vi "teleop_Moteur_Independant.vi"(11 "SwerveDrive":T1) -> ()   [LabVIEW 2018]
doc: "Les axes X and Y sont les deux axes qui font avancer le robot. X est horizontal et Y vertical selon le pilote.\nL'axez Z est l'axe qui permet au pilote de tourner en avançant dans une direction.\nLes boutons gauche et droite permettent au robot de tourner sur lui-même vers la gauche ou vers la droite selon quel bouton est actif.\n\nLe code vérifie que les roues sont dans le bon angle avant de faire avancer le robot."
uses:
  SwerveDrive.ctl
  <vilib>/addons/control/pid/pid.llb/PID (DBL).vi
  MyGlobal.vi
  <vilib>/addons/control/pid/NI_PID_pid.lvlib
panel:
  out "OUTPUT avant gauche":dbl format="%.2f"
  out "result":bool
  out "Encodeur angle arriere droite":bool
  out "Encodeur angle arriere gauche":bool
  out "Encodeur angle arriere droite":dbl
  out "Encodeur angle arriere gauche":dbl
  out "Encodeur angle avant droite":bool
  out "Encodeur angle avant gauche":bool
  out "angle roues":dbl
  out "Encodeur angle avant droite":dbl
  out "Encodeur angle avant gauche":dbl
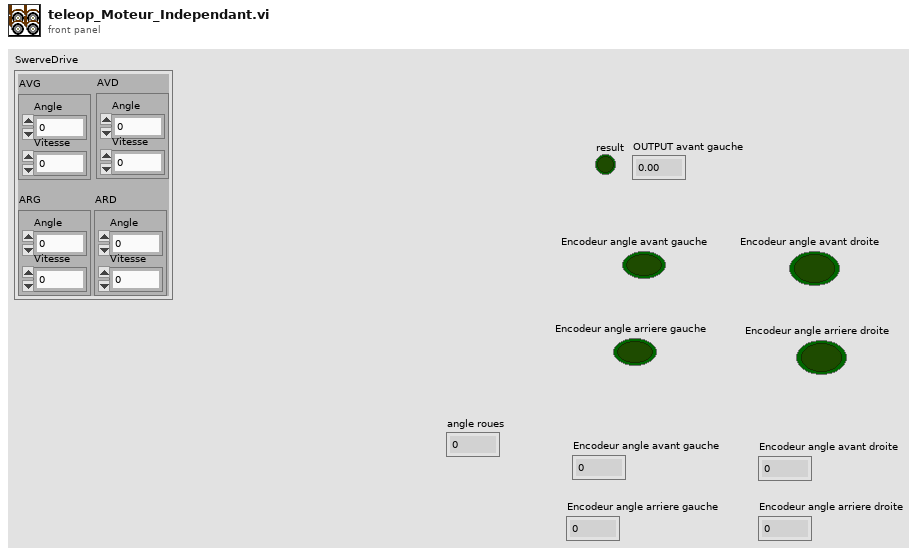
[diagram p1: front panel]
types:
  T1 = typedef "SwerveDrive.ctl" = cluster{"AVD":cluster{"Angle":dbl, "Vitesse":dbl}, "AVG":cluster{"Angle":dbl, "Vitesse":dbl}, "ARG":cluster{"Angle":dbl, "Vitesse":dbl}, "ARD":cluster{"Angle":dbl, "Vitesse":dbl}}
  T2 = cluster{"proportional gain (Kc)":dbl, "integral time (Ti, min)":dbl, "derivative time (Td, min)":dbl}
  T3 = typedef "Drivetype.ctl" = enum16{"4 vitesse", "1 vitesse"}
  T4 = typedef "WPI_MotorControlDeviceRef.ctl" = cluster{"DeviceStatus":errorcluster, "Type":T5, "PWM":cluster{"PWM Channel":T6, "DeadBand":T7}, "CAN":cluster{"Device Number":u8, "SetOutput VI Ref":variant, "GetOutput VI Ref":variant, "Enable VI Ref":variant, "Disable VI Ref":variant, "Data":variant}, "Invert":bool, "DIO PWM":cluster{"PWM \"Enable\" Channel":T6, "DIOChannel":T8, "PWM Rate":dbl}}
  T5 = typedef "WPI_MotorControlType.ctl" = enum16{"PWM", "CAN", "DIO PWM"}
  T6 = typedef "FPGA_DIOPWMChannel.ctl" = enum8{"PWM 0", "PWM 1", "PWM 2", "PWM 3", "PWM 4", "PWM 5", "PWM 6", "PWM 7", "PWM 8", "PWM 9", "PWM MXP 0", "PWM MXP 1", "PWM MXP 2", "PWM MXP 3", "PWM MXP 4", "PWM MXP 5", "PWM MXP 6", "PWM MXP 7", "PWM MXP 8", "PWM MXP 9", "Invalid"}
  T7 = typedef "WPI_PWMDeadband.ctl" = cluster{"Name":string, "maxPositivePwm":i32, "minPositivePwm":i32, "centerPwm":i32, "maxNegativePwm":i32, "minNegativePwm":i32, "angularRange":u16}
  T8 = typedef "FPGA_DIOChannel.ctl" = enum8{"DIO 0", "DIO 1", "DIO 2", "DIO 3", "DIO 4", "DIO 5", "DIO 6", "DIO 7", "DIO 8", "DIO 9", "DIO MXP 0", "DIO MXP 1", "DIO MXP 2", "DIO MXP 3", "DIO MXP 4", "DIO MXP 5", "DIO MXP 6", "DIO MXP 7", "DIO MXP 8", "DIO MXP 9", "DIO MXP 10", "DIO MXP 11", "DIO MXP 12", "DIO MXP 13", "DIO MXP 14", "DIO MXP 15", "SPI Port CS1", "SPI Port CS2", "SPI Port CS3", "SPI Port MISO", "SPI Port MOSI", "Invalid"}
  T9 = typedef "WPI_EncoderDevRef.ctl" = cluster{"DevStatus":errorcluster, "EncoderIndex":T10, "CounterIndex":T11, "DistancePerCount":dbl, "Decoding Type":T12}
  T10 = typedef "FPGA_EncoderIdx.ctl" = enum8{"Enc 0", "Enc 1", "Enc 2", "Enc 3", "Enc 4", "Enc 5", "Enc 6", "Enc 7", "Invalid"}
  T11 = typedef "FPGA_CounterCtrSystemIndex.ctl" = enum8{"Ctr 0", "Ctr 1", "Ctr 2", "Ctr 3", "Ctr 4", "Ctr 5", "Ctr 6", "Ctr 7", "Invalid"}
  T12 = typedef "WPI_EncoderType.ctl" = enum16{"1x", "2x", "4x"}
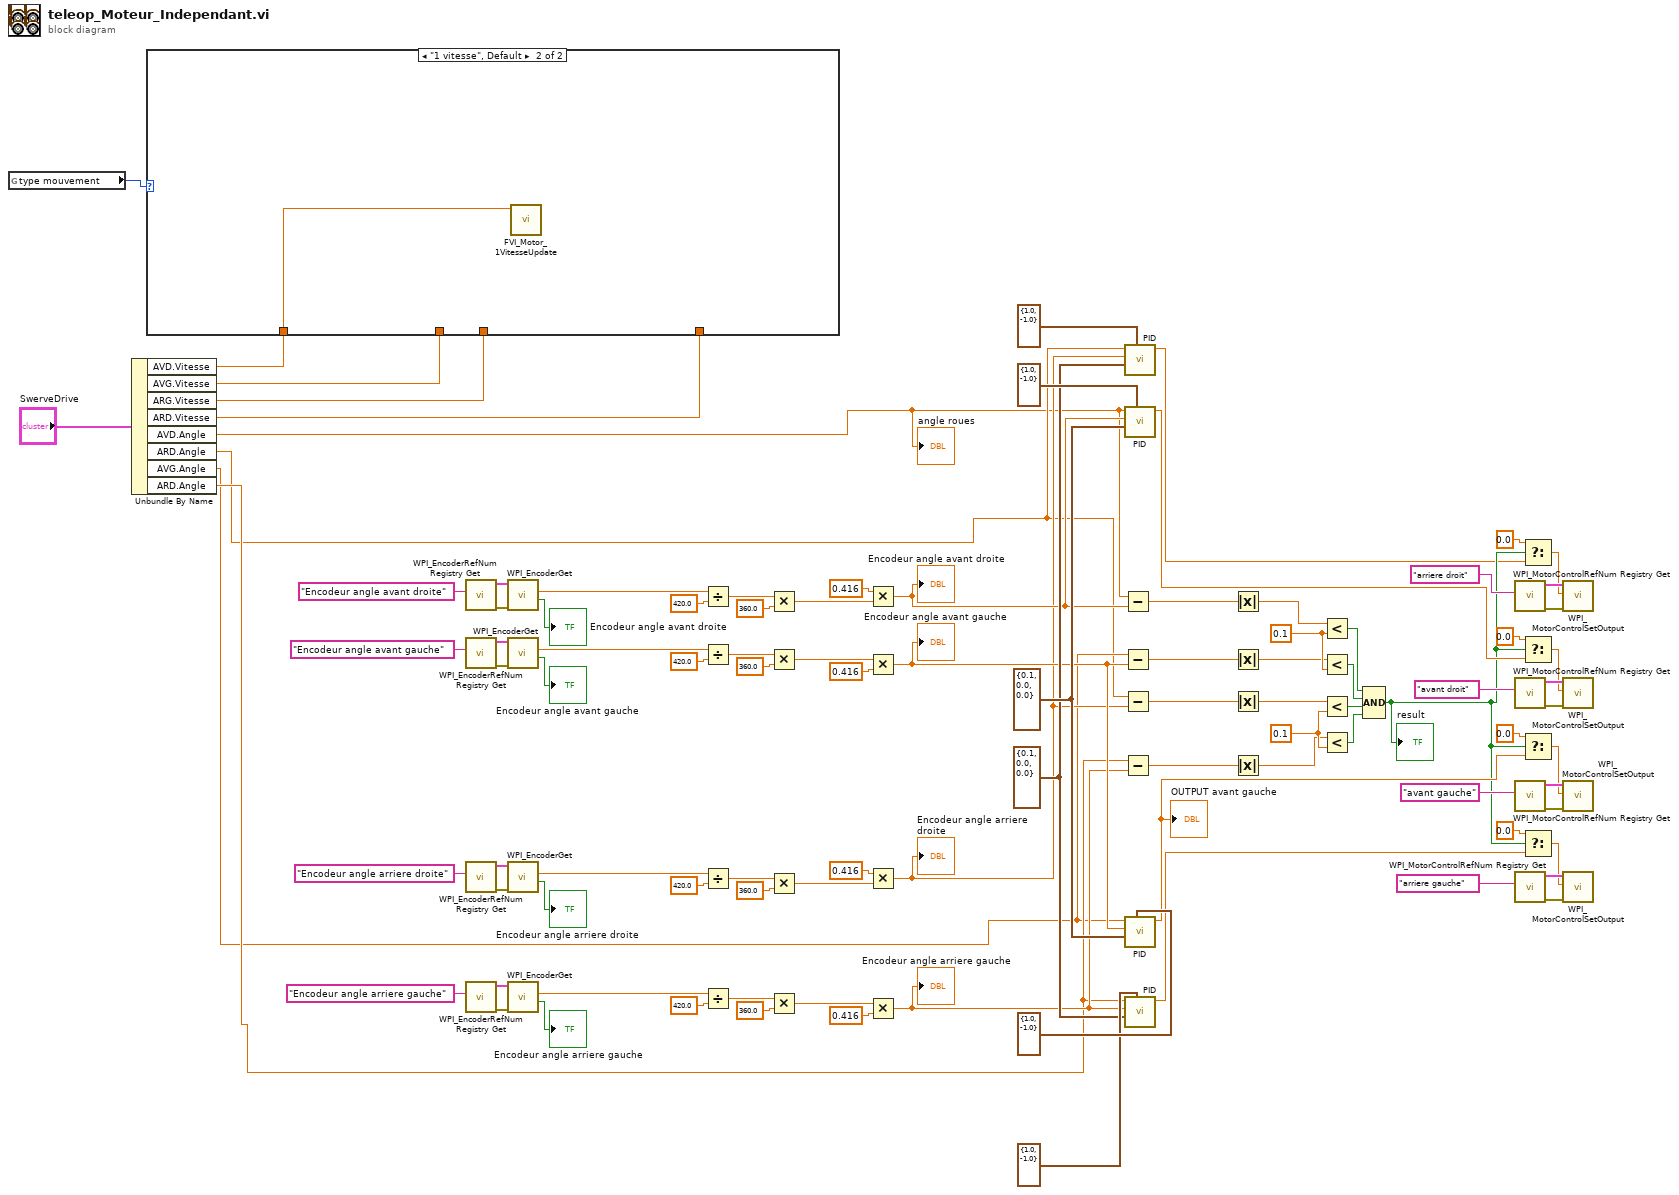
[diagram p0: block diagram]
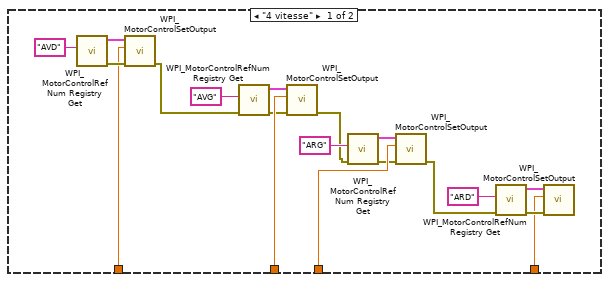
[diagram p2: hidden frame]
diagram:
  w36 = 0.1
  w35 = T2 {"proportional gain (Kc)"=0.1, "integral time (Ti, min)"=0.0, "derivative time (Td, min)"=0.0} ("PID gains")
  w63 = 0.1
  w62 = T2 {"proportional gain (Kc)"=0.1, "integral time (Ti, min)"=0.0, "derivative time (Td, min)"=0.0} ("PID gains")
  n1 = global read "MyGlobal.vi" "type mouvement"() -> (w1:T3)
  n2 = Unbundle By Name("SwerveDrive") -> ("AVD.Vitesse"=w5:dbl, "AVG.Vitesse"=w4:dbl, "ARG.Vitesse"=w3:dbl, "ARD.Vitesse"=w2:dbl, "AVD.Angle"=w6:dbl, "ARD.Angle"=w7:dbl, "AVG.Angle"=w8:dbl, "ARD.Angle"=w9:dbl)
  "angle roues" <- w6
  n3 = case shown="\"1 vitesse\", Default" w1 {
    tunnel: w5 -> [w111 w119]
    tunnel: w4 -> [w110 _]
    tunnel: w3 -> [w109 _]
    tunnel: w2 -> [w103 _]
    frame "4 vitesse" {
      n4 = call <vilib>:"WPI_MotorControlRefNum Registry Get.vi"("refnum name"="AVD") -> ("error out"=w116:errorcluster, "MotorControlDevRef"=w117:T4)  [unwired: 9 in]
      n5 = call <vilib>:"WPI_MotorControlSetOutput.vi"("error in (no error)"=w116, "Output"=w111, "MotorControlDevRef"=w117) -> ("error out"=w102:errorcluster)  [unwired: 6 in, 2 out]
      n6 = call <vilib>:"WPI_MotorControlRefNum Registry Get.vi"("error in (no error)"=w102, "refnum name"="AVG") -> ("error out"=w108:errorcluster, "MotorControlDevRef"=w115:T4)  [unwired: 8 in]
      n7 = call <vilib>:"WPI_MotorControlSetOutput.vi"("error in (no error)"=w108, "Output"=w110, "MotorControlDevRef"=w115) -> ("error out"=w101:errorcluster)  [unwired: 6 in, 2 out]
      n8 = call <vilib>:"WPI_MotorControlRefNum Registry Get.vi"("error in (no error)"=w101, "refnum name"="ARG") -> ("error out"=w107:errorcluster, "MotorControlDevRef"=w105:T4)  [unwired: 8 in]
      n9 = call <vilib>:"WPI_MotorControlSetOutput.vi"("error in (no error)"=w107, "Output"=w109, "MotorControlDevRef"=w105) -> ("error out"=w100:errorcluster)  [unwired: 6 in, 2 out]
      n10 = call <vilib>:"WPI_MotorControlRefNum Registry Get.vi"("error in (no error)"=w100, "refnum name"="ARD") -> ("error out"=w106:errorcluster, "MotorControlDevRef"=w104:T4)  [unwired: 8 in]
      n11 = call <vilib>:"WPI_MotorControlSetOutput.vi"("error in (no error)"=w106, "Output"=w103, "MotorControlDevRef"=w104) -> ()  [unwired: 6 in, 3 out]
    }
    frame "1 vitesse", Default {
      n12 = call "FVI_Motor_1VitesseUpdate.vi"("Vitesse entree"=w119) -> ()  [unwired: 10 in, 1 out]
    }
  }
  n13 = call <vilib>:"WPI_EncoderRefNum Registry Get.vi"("refnum name"="Encodeur angle avant droite") -> ("error out"=w92:errorcluster, "EncoderDevRef"=w93:T9)  [unwired: 9 in]
  n14 = call <vilib>:"WPI_EncoderRefNum Registry Get.vi"("refnum name"="Encodeur angle avant gauche") -> ("error out"=w95:errorcluster, "EncoderDevRef"=w94:T9)  [unwired: 9 in]
  n15 = call <vilib>:"WPI_EncoderRefNum Registry Get.vi"("refnum name"="Encodeur angle arriere droite") -> ("error out"=w55:errorcluster, "EncoderDevRef"=w56:T9)  [unwired: 9 in]
  n16 = call <vilib>:"WPI_EncoderRefNum Registry Get.vi"("refnum name"="Encodeur angle arriere gauche") -> ("error out"=w58:errorcluster, "EncoderDevRef"=w57:T9)  [unwired: 9 in]
  n17 = call <vilib>:"WPI_EncoderGet.vi"("error in (no error)"=w92, "EncoderDevRef"=w93) -> ("Direction"=→"Encodeur angle avant droite":bool, "Distance"=w81:dbl)  [unwired: 4 in, 4 out]
  n18 = call <vilib>:"WPI_EncoderGet.vi"("error in (no error)"=w95, "EncoderDevRef"=w94) -> ("Direction"=→"Encodeur angle avant gauche":bool, "Distance"=w80:dbl)  [unwired: 4 in, 4 out]
  n19 = call <vilib>:"WPI_EncoderGet.vi"("error in (no error)"=w55, "EncoderDevRef"=w56) -> ("Direction"=→"Encodeur angle arriere droite":bool, "Distance"=w48:dbl)  [unwired: 4 in, 4 out]
  n20 = call <vilib>:"WPI_EncoderGet.vi"("error in (no error)"=w58, "EncoderDevRef"=w57) -> ("Direction"=→"Encodeur angle arriere gauche":bool, "Distance"=w47:dbl)  [unwired: 4 in, 4 out]
  n21 = Divide(x=w81, y=420.0) -> (x/y=w84:dbl)
  n22 = Divide(x=w80, y=420.0) -> (x/y=w87:dbl)
  n23 = Divide(x=w48, y=420.0) -> (x/y=w51:dbl)
  n24 = Divide(x=w47, y=420.0) -> (x/y=w54:dbl)
  n25 = Multiply(x=w84, y=360.0) -> (x*y=w77:dbl)
  n26 = Multiply(x=w87, y=360.0) -> (x*y=w78:dbl)
  n27 = Multiply(x=w51, y=360.0) -> (x*y=w44:dbl)
  n28 = Multiply(x=w54, y=360.0) -> (x*y=w45:dbl)
  n29 = Multiply(x=0.416 ("y"), y=w77) -> (x*y=w18:dbl)
  "Encodeur angle avant droite" <- w18
  n30 = Multiply(x=w78, y=0.416) -> (x*y=w17:dbl)
  "Encodeur angle avant gauche" <- w17
  n31 = Multiply(x=0.416 ("y"), y=w44) -> (x*y=w16:dbl)
  "Encodeur angle arriere droite" <- w16
  n32 = Multiply(x=w45, y=0.416) -> (x*y=w15:dbl)
  "Encodeur angle arriere gauche" <- w15
  n33 = Subtract(x=w6, y=w18) -> (x-y=w66:dbl)
  n34 = Subtract(x=w8, y=w17) -> (x-y=w67:dbl)
  n35 = Subtract(x=w7, y=w16) -> (x-y=w39:dbl)
  n36 = Subtract(x=w9, y=w15) -> (x-y=w40:dbl)
  n37 = call-poly <vilib>:"PID.vi"("output range"=cluster{"output high":dbl, "output low":dbl} {"output high"=1.0, "output low"=-1.0}, "PID gains"=w35, "process variable"=w16, "setpoint"=w7) -> ("output"=w20:dbl)  [unwired: 6 in, 1 out]
  n38 = call-poly <vilib>:"PID.vi"("output range"=cluster{"output high":dbl, "output low":dbl} {"output high"=1.0, "output low"=-1.0}, "PID gains"=w62, "process variable"=w18, "setpoint"=w6) -> ("output"=w60:dbl)  [unwired: 6 in, 1 out]
  n39 = call-poly <vilib>:"PID.vi"("output range"=cluster{"output high":dbl, "output low":dbl} {"output high"=1.0, "output low"=-1.0}, "PID gains"=w62, "process variable"=w17, "setpoint"=w8) -> ("output"=w61:dbl)  [unwired: 6 in, 1 out]
  "OUTPUT avant gauche" <- w61
  n40 = call-poly <vilib>:"PID.vi"("output range"=cluster{"output high":dbl, "output low":dbl} {"output high"=1.0, "output low"=-1.0}, "PID gains"=w35, "process variable"=w15, "setpoint"=w9) -> ("output"=w21:dbl)  [unwired: 6 in, 1 out]
  n41 = Absolute Value(x=w66) -> (abs(x)=w14:dbl)
  n42 = Absolute Value(x=w67) -> (abs(x)=w13:dbl)
  n43 = Absolute Value(x=w39) -> (abs(x)=w12:dbl)
  n44 = Absolute Value(x=w40) -> (abs(x)=w11:dbl)
  n45 = Less?(x=w14, y=w63) -> (x < y?=w68:bool)
  n46 = Less?(x=w13, y=w63) -> (x < y?=w69:bool)
  n47 = Less?(x=w12, y=w36) -> (x < y?=w34:bool)
  n48 = Less?(x=w11, y=w36) -> (x < y?=w33:bool)
  n49 = Compound Arithmetic op=AND(w68, w69, w34, w33) -> (w22:bool)
  "result" <- w22
  n50 = call <vilib>:"WPI_MotorControlRefNum Registry Get.vi"("refnum name"="arriere droit") -> ("error out"=w30:errorcluster, "MotorControlDevRef"=w29:T4)  [unwired: 9 in]
  n51 = call <vilib>:"WPI_MotorControlRefNum Registry Get.vi"("refnum name"="avant droit") -> ("error out"=w91:errorcluster, "MotorControlDevRef"=w90:T4)  [unwired: 9 in]
  n52 = call <vilib>:"WPI_MotorControlRefNum Registry Get.vi"("refnum name"="avant gauche") -> ("error out"=w89:errorcluster, "MotorControlDevRef"=w88:T4)  [unwired: 9 in]
  n53 = call <vilib>:"WPI_MotorControlRefNum Registry Get.vi"("refnum name"="arriere gauche") -> ("error out"=w28:errorcluster, "MotorControlDevRef"=w27:T4)  [unwired: 9 in]
  n54 = Select(t=0.0 ("f"), s=w22, f=w20) -> (s? t:f=w25:dbl)
  n55 = Select(t=0.0 ("f"), s=w22, f=w60) -> (s? t:f=w73:dbl)
  n56 = Select(t=0.0 ("f"), s=w22, f=w61) -> (s? t:f=w72:dbl)
  n57 = Select(t=0.0 ("f"), s=w22, f=w21) -> (s? t:f=w24:dbl)
  n58 = call <vilib>:"WPI_MotorControlSetOutput.vi"("error in (no error)"=w30, "Output"=w25, "MotorControlDevRef"=w29) -> ()  [unwired: 6 in, 3 out]
  n59 = call <vilib>:"WPI_MotorControlSetOutput.vi"("error in (no error)"=w91, "Output"=w73, "MotorControlDevRef"=w90) -> ()  [unwired: 6 in, 3 out]
  n60 = call <vilib>:"WPI_MotorControlSetOutput.vi"("error in (no error)"=w89, "Output"=w72, "MotorControlDevRef"=w88) -> ()  [unwired: 6 in, 3 out]
  n61 = call <vilib>:"WPI_MotorControlSetOutput.vi"("error in (no error)"=w28, "Output"=w24, "MotorControlDevRef"=w27) -> ()  [unwired: 6 in, 3 out]
